vi "FTW-Actor-Tag-Get.vi"(0 "FTW-ActorInstance In":refnum<class "FTW-ActorInstance.lvclass">, 7 "Tag Object":variant, 11 "error in":errorcluster) -> (4 "FTW-ActorInstance Out":refnum<class "FTW-ActorInstance.lvclass">, 8 "Response":string, 15 "error out":errorcluster)   [LabVIEW 2015, in "FTW-ActorInstance.lvclass"]
uses:
  FTW-ActorInstance.lvclass
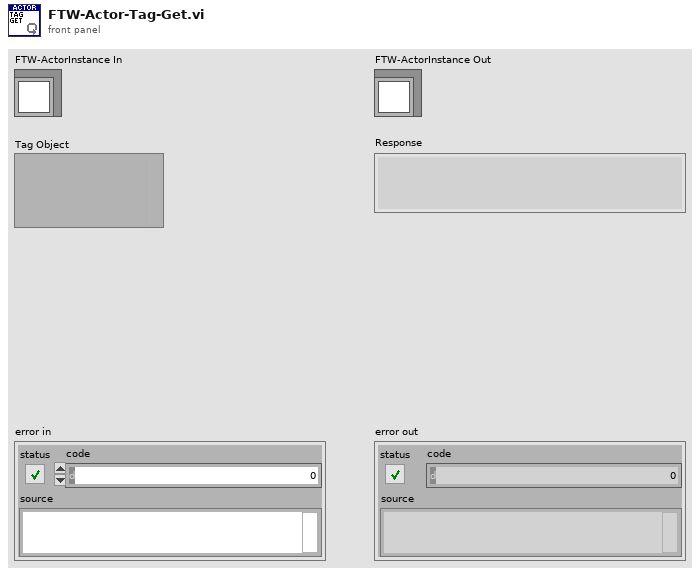
[diagram p1: front panel]
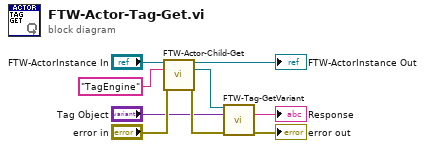
[diagram p0: block diagram]
diagram:
  n1 = call "FTW-Actor-Child-Get.vi"("FTW-ActorInstance In"="FTW-ActorInstance In", "Connector Name"="TagEngine", "error in"="error in") -> ("FTW-ActorInstance Out"=→"FTW-ActorInstance Out":refnum<class "FTW-ActorInstance.lvclass">, "FTW Actor Connector"=w7:refnum<class "FTW-ActorConnector.lvclass">, "error out"=w8:errorcluster)  [unwired: 10 in]
  n2 = call "FTW-Tag-GetVariant.vi"("FTW Actor Connector In"=w7, "Tag Object"="Tag Object", "error in (no error)"=w8) -> ("Response"=→"Response":string, "error out"=→"error out":errorcluster)  [unwired: 9 in, 2 out]
